vi "GeraComponente.vi"(0 "Amplitude":dbl, 1 "Frequencia":dbl, 2 "Fase":dbl, 3 "Tx Aquisicao":dbl) -> (15 "componente wfm":waveform(dbl), 17 "fase saida":dbl format="%0.2e")   [LabVIEW 2017]
uses:
  <vilib>/Analysis/NI_AALBase.lvlib
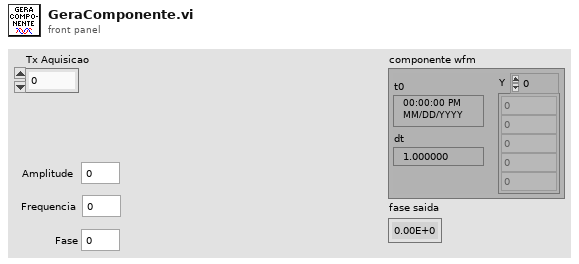
[diagram p1: front panel]
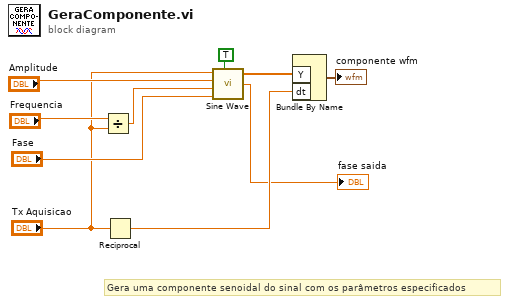
[diagram p0: block diagram]
diagram:
  # "Gera uma componente senoidal do sinal com os parâmetros especificados"
  n1 = Divide(x="Frequencia", y="Tx Aquisicao") -> (x/y=w8:dbl)
  n2 = Reciprocal(x="Tx Aquisicao") -> (1/x=w3:dbl)
  n3 = call <vilib>:"Sine Wave.vi"("samples"="Tx Aquisicao", "amplitude"="Amplitude", "frequency"=w8, "phase in"="Fase", "reset phase"=TRUE) -> ("sine wave"=w5:dbl[], "phase out"=→"fase saida":dbl)  [unwired: 1 out]
  n4 = Bundle By Name("Y"=w5, "dt"=w3) -> (→"componente wfm":waveform(dbl))  [unwired: 1 in]
